vi "Format Paths.vi"(7 "Git Implementation in":refnum<class "Git Implementation.lvclass">, 11 "File Paths":path[](array[path])) -> (3 "Formatted Path String":string)   [LabVIEW 2017, in "Git-LabVIEW.lvlib" / "Git Implementation.lvclass"]
doc: "Converts an array of paths to a string that can be used to provide a \"pathspec\" element for Git commands."
uses:
  Git Implementation.lvclass
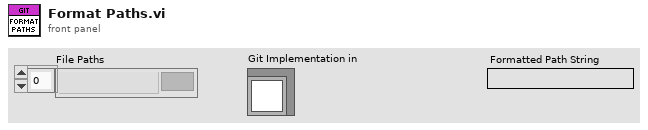
[diagram p1: front panel]
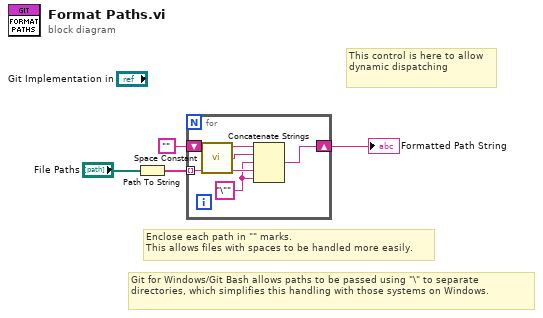
[diagram p0: block diagram]
diagram:
  # "Git for Windows/Git Bash allows paths to be passed using \"\\\" to separate directories, which simplifies this handling with those systems on Windows."
  # "Enclose each path in \"\" marks.\nThis allows files with spaces to be handled more easily."
  # "This control is here to allow dynamic dispatching"
  n1 = Path To String(path="File Paths") -> (string=w3:string[])
  n2 = for {
    tunnel: w3 -> [w9] mode=indexing
    shift-right: [w5] -> w1
    shift-left: "" -> [w7]
    w8 = "\""
    n3 = call <vilib>:"Space Constant.vi"() -> ("String"=w6:string)
    n4 = Concatenate Strings(w7, w6, w8, w9, w8) -> (w5:string)
  }
  "Formatted Path String" <- w1
